vi "Get DDG Lite Initial Delay.vi"(8 "error in (no error)":errorcluster, 10 "fDelay":sgl, 11 "channel":u32(ring)=65535 items=["AT_DDGLite_ChannelA"=1073741824, "AT_DDGLite_ChannelB"=1073741825, "AT_DDGLite_ChannelC"=1073741826]) -> (0 "error out":errorcluster, 2 "fDelay out":sgl, 3 "function return":u32)   [LabVIEW 2014, in "atmcd32d.lvlib"]
doc: "unsigned int WINAPI GetDDGLiteInitialDelay(AT_DDGLiteChannelId channel, float * fDelay);"
uses:
  atmcd32d.lvlib
  atmcd32d.dll
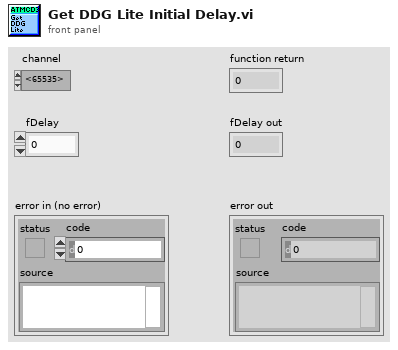
[diagram p1: front panel]
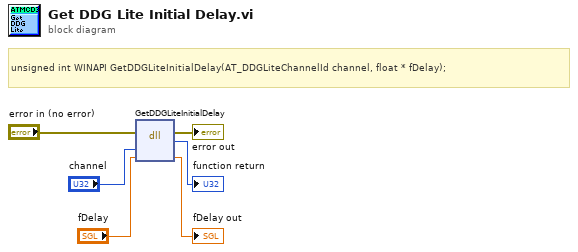
[diagram p0: block diagram]
diagram:
  # "unsigned int WINAPI GetDDGLiteInitialDelay(AT_DDGLiteChannelId channel, float * fDelay);"
  n1 = dll-call lib="C:/Users/Bakir/Documents/Lambda2-Testing/lib/Andorlib/atmcd32d.*" fn="GetDDGLiteInitialDelay"(error in="error in (no error)", "channel"="channel", "fDelay"="fDelay") -> (error out=→"error out":errorcluster, →"function return":u32, "fDelay"=→"fDelay out":sgl)  [unwired: 3 in, 1 out]
